vi "input.vi"(8 "error in":errorcluster, 10 "data table in":T1, 11 "Daqmx Module runtime in":refnum<class "DAQmx Module Runtime.lvclass">) -> (0 "error out":errorcluster, 2 "data table out":T1, 3 "Daqmx Module runtime out":refnum<class "DAQmx Module Runtime.lvclass">)   [LabVIEW 2015, in "DAQmx Module Runtime.lvclass"]
doc: "Provides an interface for reading data from a module at runtime. While this interface performs no operations, a child should provide an override which may read from any open sessions, references, or interfaces."
uses:
  DAQmx Module Runtime.lvclass
  <vilib>/NI/Tag Bus/table/data table.ctl
  DAQmx Module Runtime.lvclass/DAQmx Module Runtime.ctl
  <vilib>/DAQmx/read.llb/DAQmx Read (Analog 1D DBL NChan 1Samp).vi
  <vilib>/NI/Tag Bus/table/data polymorphs/write many/write Doubles.vi
  <vilib>/DAQmx/read.llb/DAQmx Read (Digital 1D Bool NChan 1Samp 1Line).vi
  <vilib>/NI/Tag Bus/table/data polymorphs/write many/write Booleans.vi
  <vilib>/DAQmx/miscellaneous.llb/DAQmx Fill In Error Info.vi
  <vilib>/NI/Tag Bus/table/data table.lvlib
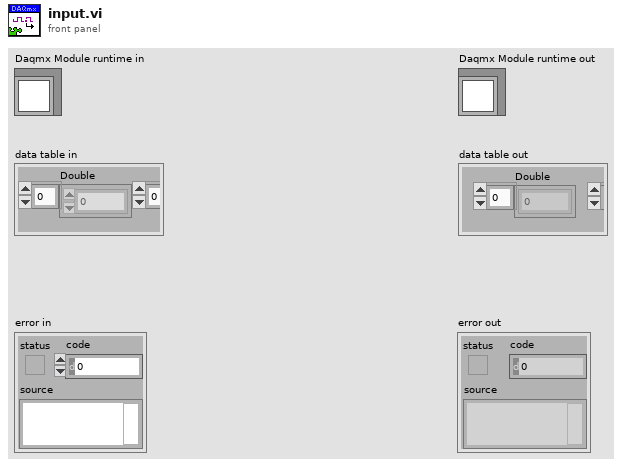
[diagram p1: front panel]
types:
  T1 = typedef "tag bus.lvlib/data table.lvlib/data table.ctl" = cluster{"Double":dbl[], "Single":sgl[], "I64":i64[], "I32":i32[], "I16":i16[], "I8":i8[], "U64":u64[], "U32":u32[], "U16":u16[], "U8":u8[], "Boolean":bool[], "String":string[], "Array of Double":cluster{"DBL Array":dbl[]}[], "Array of Single":cluster{"SGL Array":sgl[]}[], "Array of I64":cluster{"I64 Array":i64[]}[], "Array of I32":cluster{"I32 Array":i32[]}[], "Array of I16":cluster{"I16 Array":i16[]}[], "Array of I8":cluster{"I8 Array":i8[]}[], "Array of U64":cluster{"U64 Array":u64[]}[], "Array of U32":cluster{"U32 Array":u32[]}[], "Array of U16":cluster{"U16 Array":u16[]}[], "Array of U8":cluster{"U8 Array":u8[]}[], "Array of Boolean":cluster{"Boolean Array":bool[]}[], "Array of String":cluster{"String Array":string[]}[]}
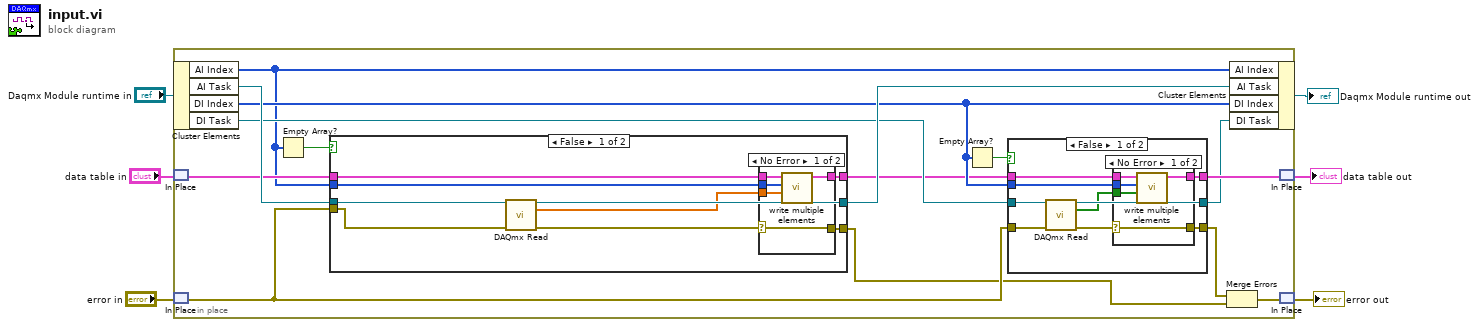
[diagram p0: block diagram]
diagram:
  n1 = in-place {
    n2 = in-place-cluster #1("Daqmx Module runtime in") -> ("AI Index"=w11:i32[], "AI Task"=w21:refnum<k21>, "DI Index"=w13:i32[], "DI Task"=w17:refnum<k21>)
    n3 = in-place-match #2("data table in") -> (w19:T1)
    n4 = in-place-match #3("error in") -> (w8:errorcluster)
    n5 = Empty Array?(array=w11) -> (empty?=w12:bool)
    n6 = case shown="False" w12 {
      tunnel: w21 -> [w42 w59]
      tunnel: [w49 w59] -> w20
      tunnel: w19 -> [w48 w57]
      tunnel: [w47 w57] -> w10
      tunnel: w8 -> [w41 w58]
      tunnel: [w44 w58] -> w7
      tunnel: w11 -> [w43 _]
      frame False {
        n7 = call-poly <vilib>:"DAQmx Read.vi"("task/channels in"=w42, "error in"=w41) -> ("task out"=w49:refnum<k21>, "data"=w46:dbl[], "error out"=w45:errorcluster)  [unwired: 11 in]
        n8 = case shown="No Error" w45 {
          selector: w45 -> [w51 w56]
          tunnel: w48 -> [w54 w55]
          tunnel: [w53 w55] -> w47
          tunnel: w46 -> [w52 _]
          tunnel: [w51 w56] -> w44
          tunnel: w43 -> [w50 _]
          frame No Error {
            n9 = call-poly <vilib>:"write multiple elements.vi"("values"=w52, "indices"=w50, "data table in"=w54) -> ("data table out"=w53:T1)  [unwired: 8 in]
          }
          frame Error {
          }
        }
      }
      frame True {
      }
    }
    n10 = Empty Array?(array=w13) -> (empty?=w14:bool)
    n11 = case shown="False" w14 {
      tunnel: w17 -> [w30 w40]
      tunnel: [w29 w40] -> w15
      tunnel: w10 -> [w28 w38]
      tunnel: [w27 w38] -> w18
      tunnel: w8 -> [w25 w39]
      tunnel: [w23 w39] -> w9
      tunnel: w13 -> [w22 _]
      frame False {
        n12 = call-poly <vilib>:"DAQmx Read.vi"("task/channels in"=w30, "error in"=w25) -> ("task out"=w29:refnum<k21>, "data"=w26:bool[], "error out"=w24:errorcluster)  [unwired: 11 in]
        n13 = case shown="No Error" w24 {
          selector: w24 -> [w32 w37]
          tunnel: w28 -> [w35 w36]
          tunnel: [w34 w36] -> w27
          tunnel: w26 -> [w33 _]
          tunnel: [w32 w37] -> w23
          tunnel: w22 -> [w31 _]
          frame No Error {
            n14 = call-poly <vilib>:"write multiple elements.vi"("values"=w33, "indices"=w31, "data table in"=w35) -> ("data table out"=w34:T1)  [unwired: 8 in]
          }
          frame Error {
          }
        }
      }
      frame True {
      }
    }
    n15 = Merge Errors(w9, w7) -> (w16:errorcluster)
    n16 = in-place-cluster #1("AI Index"=w11, "AI Task"=w20, "DI Index"=w13, "DI Task"=w15) -> (→"Daqmx Module runtime out":refnum<class "DAQmx Module Runtime.lvclass">)
    n17 = in-place-match #2(w18) -> (→"data table out":T1)
    n18 = in-place-match #3(w16) -> (→"error out":errorcluster)
  }
